vi "FMPA LogSort_StackHandler.vi"(2 "Indices":cluster{"First":i32, "Last":i32}, 6 "split":i32) -> (18 "Stacked?":bool)   [LabVIEW 2023]
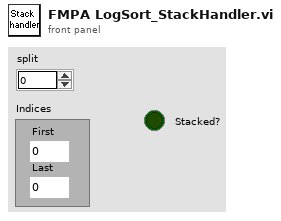
[diagram p1: front panel]
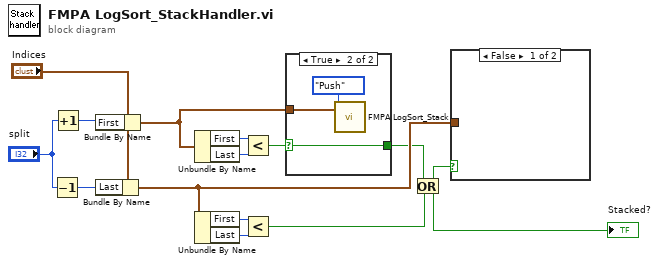
[diagram p0: block diagram]
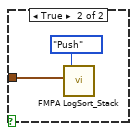
[diagram p2: hidden frame]
diagram:
  n1 = Decrement(x="split") -> (x-1=w14:i32)
  n2 = Increment(x="split") -> (x+1=w13:i32)
  n3 = Bundle By Name(cluster="Indices", "First"=w13) -> (w11:cluster{"First":i32, "Last":i32})
  n4 = Bundle By Name(cluster="Indices", "Last"=w14) -> (w10:cluster{"First":i32, "Last":i32})
  n5 = Unbundle By Name(w11) -> ("First"=w9:i32, "Last"=w8:i32)
  n6 = Unbundle By Name(w10) -> ("First"=w7:i32, "Last"=w6:i32)
  n7 = Less?(x=w9, y=w8) -> (x < y?=w4:bool)
  n8 = Less?(x=w7, y=w6) -> (x < y?=w5:bool)
  n9 = case shown="True" w4 {
    selector: w4 -> [w15 w16]
    tunnel: w11 -> [_ w18]
    tunnel: [w15 w16] -> w3
    frame False {
    }
    frame True {
      n10 = call "FMPA LogSort_Stack.vi"("Function"=enum16{"Init", "Push", "Pop", "Size"}."Push", "Indices"=w18) -> ()  [unwired: 16 in, 2 out]
    }
  }
  n11 = Or(x=w3, y=w5) -> (x .or. y?=w2:bool)
  "Stacked?" <- w2
  n12 = case shown="False" w2 {
    tunnel: w10 -> [_ w20]
    frame False {
    }
    frame True {
      n13 = call "FMPA LogSort_Stack.vi"("Function"=enum16{"Init", "Push", "Pop", "Size"}."Push", "Indices"=w20) -> ()  [unwired: 16 in, 2 out]
    }
  }
